vi "Gyro Read.vi"(8 "error in (no error)":errorcluster, 11 "I2CDevRef In":T2={"DevStatus"={"status"=FALSE, "code"=0, "source"=""}, "Controller"=enum."Controller 1", "Device Address"=0, "Handle"=0, "I2C Bus"=enum."Invalid"} {"Device Address" format="%.0x"}) -> (0 "error out":errorcluster, 2 "Angular Rate":dbl, 3 "Angle":dbl)   [LabVIEW 2014]
uses:
  <vilib>/Rock Robotics/WPI/I2C/WPI_I2CDevRef.ctl
  <vilib>/Rock Robotics/SystemInterfaces/Typedef/FPGA_TypedefDigitalModule.ctl
  <vilib>/Rock Robotics/SystemInterfaces/i2clib/i2c_bus.ctl
  DPS Mode.ctl
  Gyro Globals.vi
panel:
  out "Current Field Angle":dbl(graph)
  out "DPS Mode":T1
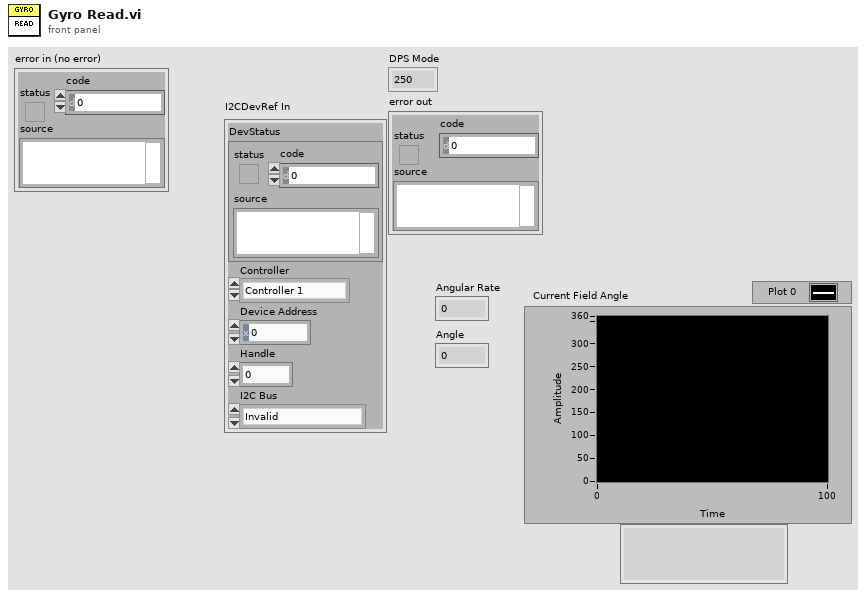
[diagram p1: front panel]
types:
  T1 = typedef "DPS Mode.ctl" = enum16{"250", "500", "2000"}
  T2 = typedef "WPI_I2CDevRef.ctl" = cluster{"DevStatus":errorcluster, "Controller":T3, "Device Address":u8, "Handle":i32, "I2C Bus":T4}
  T3 = typedef "FPGA_TypedefDigitalModule.ctl" = enum16{"Controller 1"}
  T4 = typedef "i2c_bus.ctl" = enum16{"I2C On-Board", "I2C MXP", "Invalid"}
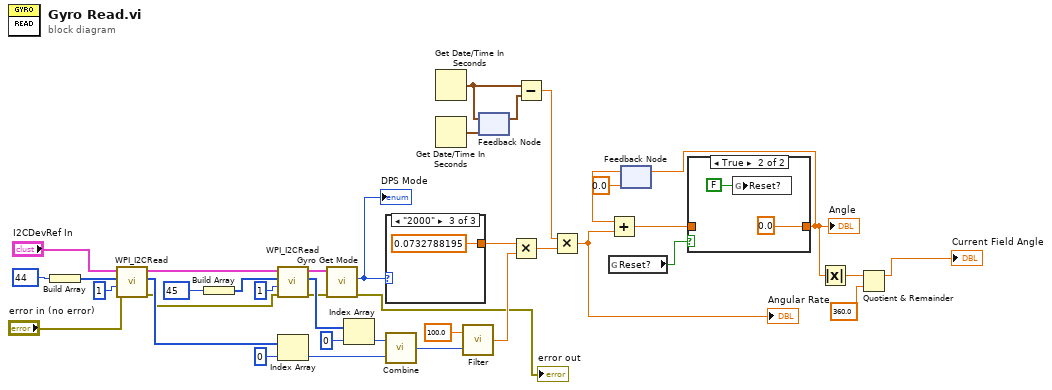
[diagram p0: block diagram]
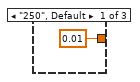
[diagram p3: hidden frame]
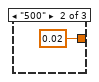
[diagram p4: hidden frame]
diagram:
  n1 = Build Array(u8 44 ("Data To Send")) -> (w38:u8[])
  n2 = call <vilib>:"WPI_I2CRead.vi"("error in (no error)"="error in (no error)", "I2CBytesToRead"=u8 1, "I2CRegister"=w38, "I2CDevRef"="I2CDevRef In") -> ("error out"=w8:errorcluster, "Data Out"=w31:u8[], "I2CDevRef"=w32:T2)  [unwired: 5 in]
  n3 = Build Array(u8 45 ("Data To Send")) -> (w34:u8[])
  n4 = call <vilib>:"WPI_I2CRead.vi"("error in (no error)"=w8, "I2CBytesToRead"=u8 1, "I2CRegister"=w34, "I2CDevRef"=w32) -> ("error out"=w7:errorcluster, "Data Out"=w28:u8[], "I2CDevRef"=w17:T2)  [unwired: 5 in]
  n5 = Index Array(array=w31, index=0) -> (element=w26:u8)
  n6 = call "Gyro Get Mode.vi"("error in (no error)"=w7, "I2CDevRef"=w17) -> ("error out"=→"error out":errorcluster, "DPS Mode"=w16:T1)  [unwired: 7 in, 1 out]
  "DPS Mode" <- w16
  n7 = Index Array(array=w28, index=0) -> (element=w27:u8)
  n8 = case shown="\"2000\"" w16 {
    tunnel: [0.01 ("Gyro Gain") 0.02 ("Gyro Gain") 0.0732788195 ("Gyro Gain")] -> w15
    frame "250", Default {
    }
    frame "500" {
    }
    frame "2000" {
    }
  }
  n9 = call "Combine.vi"("L"=w26, "H"=w27) -> ("Out"=w25:i16)
  n10 = Get Date/Time In Seconds() -> (seconds since 1Jan1904=w11:timestamp)
  n11 = Get Date/Time In Seconds() -> (seconds since 1Jan1904=w10:timestamp)
  n12 = call "Filter.vi"("In"=w25, "Window"=100.0) -> ("Out"=w22:dbl)
  n13 = feedback-in #1(w11) -> ()
  n14 = feedback #1(w10) -> (w12:timestamp)
  n15 = Multiply(x=w15, y=w22) -> (x*y=w23:dbl)
  n16 = Subtract(x=w11, y=w12) -> (x-y=w9:dbl)
  n17 = Multiply(x=w9, y=w23) -> (x*y=w20:dbl)
  "Angular Rate" <- w20
  n18 = global read "Gyro Globals.vi" "Reset?"() -> (w14:bool)
  n19 = feedback #2(0.0) -> (w19:dbl)
  n20 = Add(x=w19, y=w20) -> (x+y=w13:dbl)
  n21 = case shown="True" w14 {
    tunnel: w13 -> [w42 _]
    tunnel: [w42 0.0] -> w3
    frame False {
    }
    frame True {
      n22 = global write "Gyro Globals.vi" "Reset?"(FALSE ("Reset?")) -> ()
    }
  }
  "Angle" <- w3
  n23 = feedback-in #2(w3) -> ()
  n24 = Absolute Value(x=w3) -> (abs(x)=w4:dbl)
  n25 = Quotient & Remainder(x=w4, y=360.0) -> (x-y*floor(x/y)=→"Current Field Angle":dbl)  [unwired: 1 out]
